vi "GetParam.vi"(8 "error in (no error)":errorcluster caption="entrée d'erreur (pas d'erreur)", 11 "Nystroem.lvclass":refnum<class "Nystroem.lvclass">) -> (0 "error out":errorcluster caption="sortie d'erreur", 2 "Nystroem":T1={"kernel"="rbf", "gamma"="None", "coef0"="None", "degree"="None", "kernel_params"="None", "n_components"=100, "random_state"=-1} {"random_state" min=-1}, 3 "Nystroem.lvclass":refnum<class "Nystroem.lvclass">)   [LabVIEW 2020, in "Nystroem.lvclass"]
doc: "Get Parameters"
uses:
  Nystroem.lvclass
  Nystroem.lvclass/Nystroem.ctl
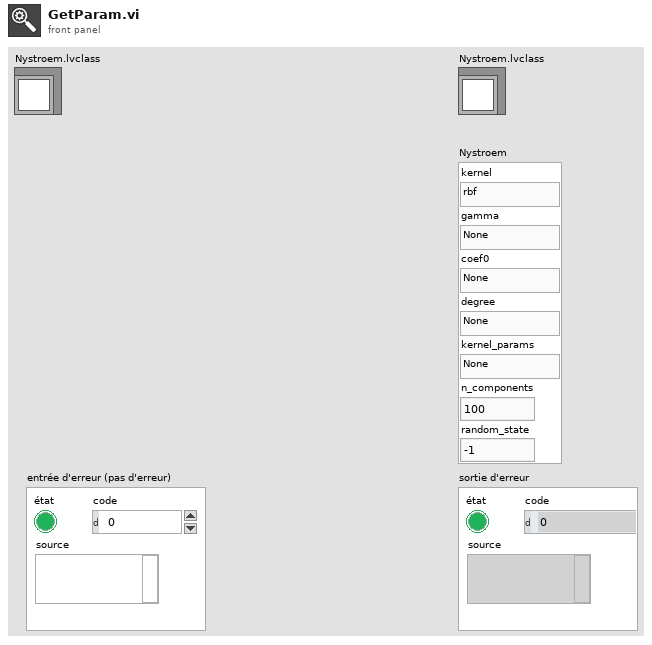
[diagram p1: front panel]
types:
  T1 = cluster{"kernel":string, "gamma":string, "coef0":string, "degree":string, "kernel_params":string, "n_components":i32, "random_state":i32}
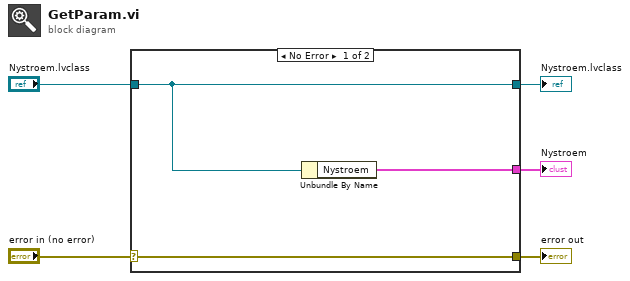
[diagram p0: block diagram]
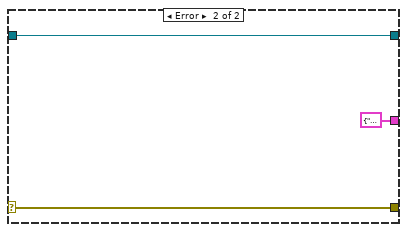
[diagram p2: hidden frame]
diagram:
  n1 = case shown="No Error" "error in (no error)" {
    selector: "error in (no error)" -> [w8 w10]
    tunnel: [w8 w10] -> w4
    tunnel: [w7 w11] -> w2
    tunnel: "Nystroem.lvclass" -> [w7 w11]
    tunnel: [w6 T1 {"kernel"="", "gamma"="", "coef0"="", "degree"="", "kernel_params"="", "n_components"=0, "random_state"=0} ("Nystroem")] -> w1
    frame No Error {
      n2 = Unbundle By Name(w7) -> ("Nystroem"=w6:T1)
    }
    frame Error {
    }
  }
  "error out" <- w4
  "Nystroem.lvclass" <- w2
  "Nystroem" <- w1
